vi "Init.vi"(8 "error in (no error)":errorcluster, 10 "Instrument String":variant, 11 "NI Scope in":refnum<class "NI Scope.lvclass">) -> (0 "error out":errorcluster, 2 "Found?":bool=TRUE, 3 "NI Scope out":refnum<class "NI Scope.lvclass">)   [LabVIEW 2025, in "Scope.lvlib" / "NI Scope.lvclass"]
uses:
  NI Scope.lvclass
  C:/Working copy/tss/Plugin/Engines/Scope/Scope Instrument/Scope Instrument.lvclass
  Scope configuration/Scope configuration.lvclass
  C:/Users/Public/Documents/Sandia National Labs/TSS Plugin/Abstract Engine.lvlibp/Instrument configuration/Instrument configuration.lvclass
  NI Scope.lvclass/NI Scope.ctl
  Users/Public/Documents/Sandia National Labs/TSS Plugin/Abstract Engine.lvlibp/Instrument configuration/Read Instrument Setting.vi
  Users/Public/Documents/Sandia National Labs/TSS Plugin/CEF.lvlibp/serializable configuration/CEF_serializable configuration.lvclass
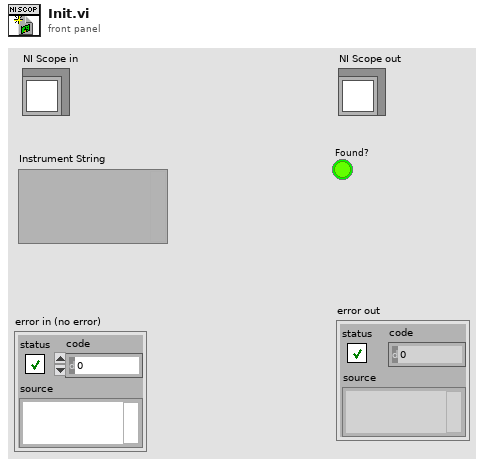
[diagram p1: front panel]
types:
  T1 = typedef "Abstract Engine.lvlibp/Instrument configuration.lvclass/Default Instrument.ctl" = cluster{"Type":string, "Address":string, "SW Alias":string, "Description":string, "Enabled":bool}
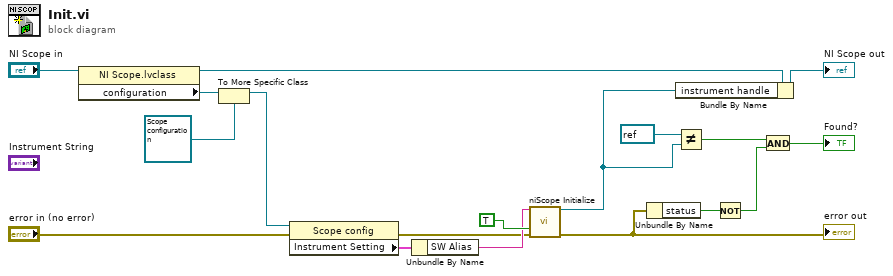
[diagram p0: block diagram]
diagram:
  n1 = property class="NI Scope.lvclass"(reference="NI Scope in") -> (reference out=w1:refnum<class "NI Scope.lvclass">, "configuration"=w11:refnum<class "CEF_serializable configuration.lvclass">)  [unwired: 1 in, 1 out]
  n2 = To More Specific Class(target class=refnum<class "Scope configuration.lvclass"> refnum ("Scope.lvlib:Scope configuration.lvclass"), reference=w11) -> (specific class reference=w10:refnum<class "Scope configuration.lvclass">)  [unwired: 1 in, 1 out]
  n3 = property class="Scope config"(reference=w10, error in="error in (no error)") -> (error out=w2:errorcluster, "Instrument Setting"=w12:T1)  [unwired: 1 out]
  n4 = Unbundle By Name(w12) -> ("SW Alias"=w14:string)
  n5 = call <instrlib>:"niScope Initialize.vi"("resource name"=w14, "reset device"=TRUE, "error in"=w2) -> ("instrument handle"=w16:refnum<k15>, "error out"=w8:errorcluster)  [unwired: 11 in]
  "error out" <- w8
  n6 = Unbundle By Name(w8) -> ("status"=w6:bool)
  n7 = Bundle By Name(cluster=w1, "instrument handle"=w16) -> (→"NI Scope out":refnum<class "NI Scope.lvclass">)
  n8 = Not Equal?(x=refnum<k15> refnum, y=w16) -> (x != y?=w7:bool)
  n9 = Not(x=w6) -> (.not. x?=w4:bool)
  n10 = And(x=w7, y=w4) -> (x .and. y?=→"Found?":bool)
